vi "Configure Session.vi"(8 "error in":errorcluster, 11 "Plugin in":refnum<class "Test Sequencer.lvclass">) -> (0 "error out":errorcluster, 3 "Plugin out":refnum<class "Test Sequencer.lvclass">)   [LabVIEW 2023, in "Test Sequencer.lvlib" / "Test Sequencer.lvclass"]
uses:
  Test Sequencer.lvclass
  C:/Program Files/National Instruments/LabVIEW 2023/vi.lib/FlexLogger/SDK/PluginSDK.lvlibp/PEFClasses/SDK/Plugin/Plugin.lvclass
  Test Sequencer.lvclass/Test Sequencer.ctl
  <vilib>/FlexLogger/SDK/PluginSDK.lvlibp/PEFClasses/SDK/Plugin/ParameterAccess/Read I32.vi
  <vilib>/FlexLogger/SDK/PluginSDK.lvlibp/PEFClasses/SDK/Plugin/ParameterAccess/Read DBL.vi
  <vilib>/FlexLogger/SDK/PluginSDK.lvlibp/PEFClasses/SDK/Plugin/ParameterAccess/Write DBL.vi
  <vilib>/FlexLogger/SDK/PluginSDK.lvlibp/PEFClasses/SDK/Plugin/ParameterAccess/Read Boolean.vi
  <vilib>/FlexLogger/SDK/PluginSDK.lvlibp/PEFClasses/SDK/Plugin/Plugin.lvclass
  C:/Program Files/National Instruments/LabVIEW 2023/vi.lib/FlexLogger/SDK/PluginSDK.lvlibp/PEFClasses/SDK/Processing Element/Processing Element.lvclass
  C:/Users/bbuchana/Documents/LabVIEW Projects/FlexLogger IO Plug-ins/Test Sequencer/Test Sequencer.lvclass
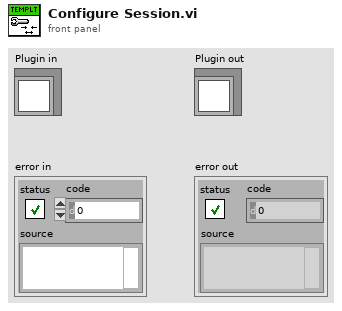
[diagram p1: front panel]
types:
  T1 = typedef "Params.ctl" = cluster{"Sequence Durations":dbl[], "Reset on Test Start":bool, "Current Sequence ID":u32, "Total Iterations":u32, "Last Timestamp":timestamp, "Number of Sequence Steps":i32}
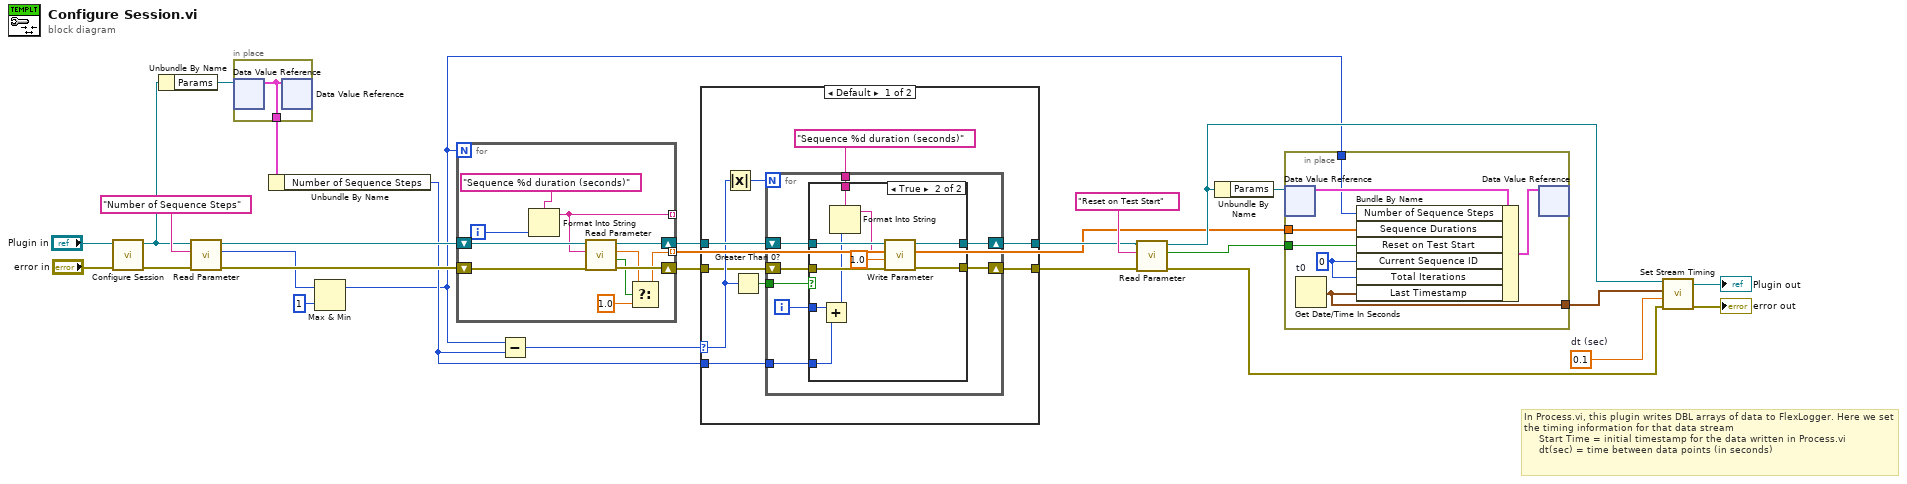
[diagram p0: block diagram]
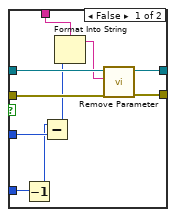
[diagram p2: hidden frame]
diagram:
  w22 = 0.1  # dt (sec)
  # "In Process.vi, this plugin writes DBL arrays of data to FlexLogger. Here we set the timing information for that data stream\n     Start Time = initial timestamp for the data written in Process.vi\n     dt(sec) = time between data points (in seconds)"
  n1 = call-parent "Configure Session.vi"("error in (no error)"="error in", "Processing Element in"="Plugin in") -> ("error out"=w17:errorcluster, "Processing Element out"=w15:refnum<class "Test Sequencer.lvclass">)  [unwired: 8 in]
  n2 = Unbundle By Name(w15) -> ("Params"=w14:refnum<data-value>)
  n3 = call-poly <vilib>:"Read Parameter.vi"("error in (no error)"=w17, "Name"="Number of Sequence Steps", "Plugin in"=w15) -> ("error out"=w11:errorcluster, "Value"=w10:i32, "Plugin out"=w12:refnum<class "Test Sequencer.lvclass">)  [unwired: 5 in, 1 out]
  n4 = in-place {
    in-place-border: [w29] -> w13
    n5 = in-place-dvr #1(w14) -> (w29:T1)  [unwired: 1 out]
    n6 = in-place-dvr #1(w29) -> ()  [unwired: 2 out]
  }
  n7 = Unbundle By Name(w13) -> ("Number of Sequence Steps"=w3:i32)
  n8 = Max & Min(x=w10, y=1) -> (max(x,y)=w1:i32)  [unwired: 1 out]
  n9 = for {
    N: w1 -> [_]
    shift-right: [w37] -> w8
    shift-left: w12 -> [w39]
    shift-right: [w36] -> w4
    shift-left: w11 -> [w38]
    tunnel: [w30] -> w6 mode=indexing
    tunnel: [w34] -> _ mode=indexing
    i -> [w35]
    n10 = Format Into String(format string="Sequence %d duration (seconds)" ("Name"), w35) -> (resulting string=w34:string)  [unwired: 2 in, 1 out]
    n11 = call-poly <vilib>:"Read Parameter.vi"("error in (no error)"=w38, "Name"=w34, "Plugin in"=w39) -> ("error out"=w36:errorcluster, "Found"=w33:bool, "Value"=w32:dbl, "Plugin out"=w37:refnum<class "Test Sequencer.lvclass">)  [unwired: 5 in]
    n12 = Select(t=w32, s=w33, f=1.0) -> (s? t:f=w30:dbl)
  }
  n13 = Subtract(x=w1, y=w3) -> (x-y=w5:i32)
  n14 = case shown="Default" w5 {
    selector: w5 -> [w47 _]
    tunnel: w8 -> [w49 w79]
    tunnel: [w42 w79] -> w7
    tunnel: w4 -> [w45 w78]
    tunnel: w3 -> [w43 _]
    tunnel: [w41 w78] -> w2
    frame Default {
      n15 = Absolute Value(x=w47) -> (abs(x)=w48:i32)
      n16 = Greater Than 0?(x=w47) -> (x > 0?=w46:bool)
      n17 = for {
        N: w48 -> [_]
        shift-right: [w56] -> w42
        shift-left: w49 -> [w57]
        tunnel: w46 -> [w55]
        shift-right: [w53] -> w41
        shift-left: w45 -> [w54]
        tunnel: "Sequence %d duration (seconds)" ("Name") -> [w52]
        tunnel: w43 -> [w50]
        i -> [w51]
        n18 = case shown="True" w55 {
          tunnel: w57 -> [w67 w77]
          tunnel: [w66 w76] -> w56
          tunnel: w54 -> [w65 w75]
          tunnel: [w64 w74] -> w53
          tunnel: w52 -> [w63 w73]
          tunnel: w51 -> [w62 w71]
          tunnel: w50 -> [w61 w70]
          frame False {
            n19 = Decrement(x=w61) -> (x-1=w60:i32)
            n20 = Subtract(x=w60, y=w62) -> (x-y=w59:i32)
            n21 = Format Into String(format string=w63, w59) -> (resulting string=w58:string)  [unwired: 2 in, 1 out]
            n22 = call <vilib>:"Remove Parameter.vi"("error in (no error)"=w65, "Name"=w58, "Plugin in"=w67) -> ("error out"=w64:errorcluster, "Plugin out"=w66:refnum<class "Test Sequencer.lvclass">)  [unwired: 7 in]
          }
          frame True {
            n23 = Add(x=w71, y=w70) -> (x+y=w69:i32)
            n24 = Format Into String(format string=w73, w69) -> (resulting string=w72:string)  [unwired: 2 in, 1 out]
            n25 = call-poly <vilib>:"Write Parameter.vi"("error in (no error)"=w75, "Value"=1.0, "Name"=w72, "Plugin in"=w77) -> ("error out"=w74:errorcluster, "Plugin out"=w76:refnum<class "Test Sequencer.lvclass">)  [unwired: 6 in]
          }
        }
      }
    }
    frame 0 {
    }
  }
  n26 = call-poly <vilib>:"Read Parameter.vi"("error in (no error)"=w2, "Name"="Reset on Test Start", "Plugin in"=w7) -> ("error out"=w23:errorcluster, "Value"=w19:bool, "Plugin out"=w24:refnum<class "Test Sequencer.lvclass">)  [unwired: 5 in, 1 out]
  n27 = Unbundle By Name(w24) -> ("Params"=w20:refnum<data-value>)
  n28 = in-place {
    in-place-border: w6 -> [w84]
    in-place-border: w19 -> [w83]
    in-place-border: [w81] -> w18
    in-place-border: w1 -> [w80]
    w82 = u32 0 ("Current Sequence ID")
    n29 = in-place-dvr #2(w20) -> (w86:T1)  [unwired: 1 out]
    n30 = Get Date/Time In Seconds "t0"() -> (seconds since 1Jan1904=w81:timestamp)
    n31 = Bundle By Name(cluster=w86, "Number of Sequence Steps"=w80, "Sequence Durations"=w84, "Reset on Test Start"=w83, "Current Sequence ID"=w82, "Total Iterations"=w82, "Last Timestamp"=w81) -> (w85:T1)
    n32 = in-place-dvr #2(w85) -> ()  [unwired: 2 out]
  }
  n33 = call-dynamic "Set Stream Timing.vi"("error in (no error)"=w23, "dt(sec)"=w22, "Start Time"=w18, "Plugin in"=w24) -> ("error out"=→"error out":errorcluster, "Plugin out"=→"Plugin out":refnum<class "Test Sequencer.lvclass">)  [unwired: 6 in]
